vi "Queue Self.vi"(9 "Priority?":bool, 10 "Msg":refnum<class "Msg.lvclass">, 11 "jettl Event Actor in":refnum<class "jettl Event Actor.lvclass">) -> (3 "jettl Event Actor out":refnum<class "jettl Event Actor.lvclass">)   [LabVIEW 2021, in "jettl.lvlib" / "jettl Event Actor.lvclass"]
uses:
  jettl Event Actor.lvclass
  Actor/Msg/Msg.lvclass
  jettl Event Actor.lvclass/jettl Event Actor.ctl
  jettl.lvlib
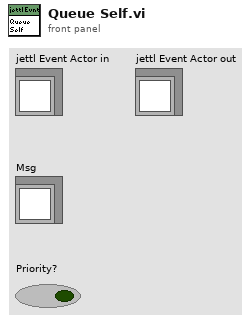
[diagram p1: front panel]
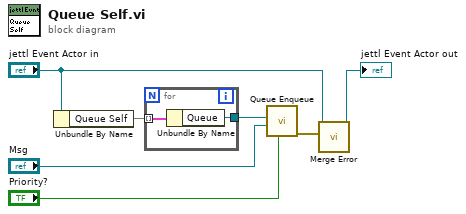
[diagram p0: block diagram]
diagram:
  n1 = Unbundle By Name("jettl Event Actor in") -> ("Queue Self"=w5:map{string, refnum<data-value>})
  n2 = for {
    tunnel: [w8] -> w6
    tunnel: w5 -> [w9] mode=indexing
    n3 = Unbundle By Name(w9) -> ("Queue"=w8:refnum<data-value>)
  }
  n4 = call "Queue Enqueue.vi"("Priority?"="Priority?", "Msg"="Msg", "Queue"=w6) -> ("error out"=w7:errorcluster)  [unwired: 8 in]
  n5 = call-dynamic "Merge Error.vi"("Error"=w7, "Set Error in"="jettl Event Actor in") -> ("Set Error out"=→"jettl Event Actor out":refnum<class "jettl Event Actor.lvclass">)  [unwired: 9 in]
